vi "ContinuousStrobeSample.vi"() -> ()   [LabVIEW 2015]
panel:
  in  "Continuous \nStrobe Delay":i32
  out "Spectrum of the first Spectrometer":cluster{"Y":dbl[], "Y":dbl[]}[](graph)
  in  "stop":bool
  in  "Enter the \nInetegration Time":i32
  in  "Start":bool=TRUE
  out "Number of Spectrometers":i32
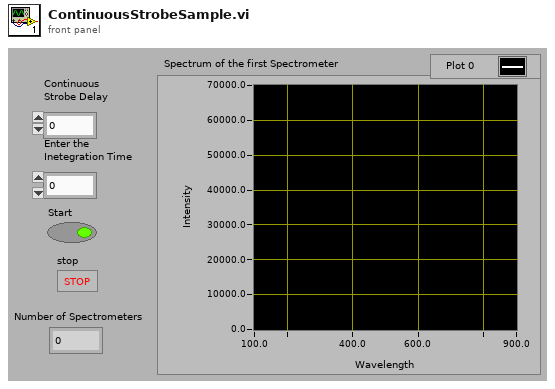
[diagram p1: front panel]
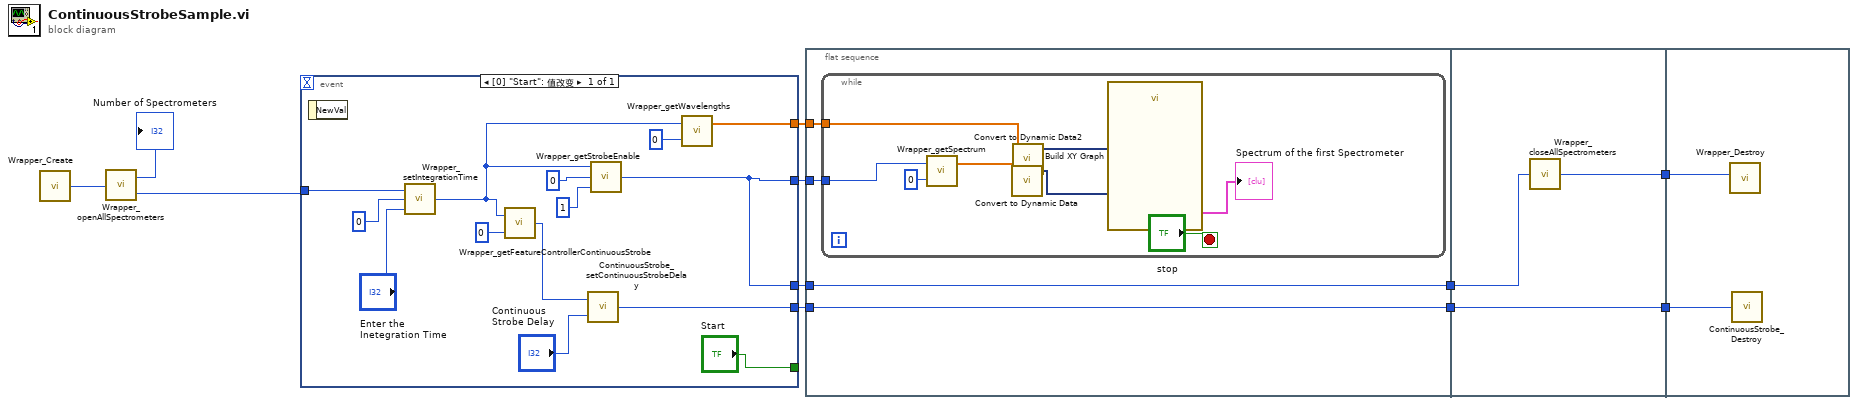
[diagram p0: block diagram]
diagram:
  n1 = call "Wrapper_Create.vi"() -> ("Wrapper"=w2:u32)
  n2 = call "Wrapper_openAllSpectrometers.vi"("Wrapper In"=w2) -> ("Number of Spectrometers"=→"Number of Spectrometers":i32, "Wrapper Out"=w1:u32)
  n3 = event shown="[0] \"Start\": 值改变" {
    selector: _ -> [_]
    dyn-events: _ -> [_]
    timeout: _ -> [_]
    tunnel: ["Start"] -> _
    tunnel: w1 -> [w22]
    tunnel: [w13] -> w10
    tunnel: [w21] -> w9
    tunnel: [w13] -> w7
    tunnel: [w12] -> w3
    event "Start": Value Change {
      n4 = event-data() -> ()  [unwired: 1 in, 1 out]
      n5 = call "Wrapper_setIntegrationTime.vi"("Integration Time"="Enter the \nInetegration Time", "Index"=0, "Wrapper In"=w22) -> ("Wrapper Out"=w16:u32)
      n6 = call "Wrapper_getFeatureControllerContinuousStrobe.vi"("Index"=0, "Wrapper"=w16) -> ("ContinuousStrobe"=w18:u32)
      n7 = call "ContinuousStrobe_setContinuousStrobeDelay.vi"("delay"="Continuous \nStrobe Delay", "ContinuousStrobe In"=w18) -> ("ContinuousStrobe Out"=w12:u32)
      n8 = call "Wrapper_getStrobeEnable.vi"("On/Off"=1, "Index"=0, "Wrapper In"=w16) -> ("Wrapper Out"=w13:u32)
      n9 = call "Wrapper_getWavelengths.vi"("Index"=0, "Wrapper"=w16) -> ("WL Values"=w21:dbl[])  [unwired: 1 out]
    }
  }
  n10 = flat-sequence {
    tunnel: w10 -> [w29]
    tunnel: w9 -> [w28]
    tunnel: [w27] -> w8
    tunnel: w7 -> [w27]
    tunnel: [w26] -> w4
    tunnel: w3 -> [w26]
    tunnel: w8 -> [w40]
    tunnel: [w39] -> w6
    tunnel: [w38] -> w5
    tunnel: w4 -> [w38]
    tunnel: w6 -> [w42]
    tunnel: w5 -> [w41]
    frame #0 {
      n11 = while {
        tunnel: w29 -> [w37]
        tunnel: w28 -> [w31]
        stop <- "stop" stop-if-true
        n12 = call "Wrapper_getSpectrum.vi"("Index"=0, "Wrapper"=w37) -> ("Spectrum Values"=w33:dbl[])  [unwired: 1 out]
        n13 = call "Convert to Dynamic Data"("Array"=w33) -> ("Dynamic Data Type"=w32:dynamicdata)  [unwired: 3 in]
        n14 = call "Convert to Dynamic Data2"("Array"=w31) -> ("Dynamic Data Type"=w30:dynamicdata)  [unwired: 3 in]
        n15 = call "Build XY Graph"("Y Input"=w32, "X Input"=w30) -> ("XY Graph"=→"Spectrum of the first Spectrometer":cluster{"Y":dbl[], "Y":dbl[]}[])  [unwired: 8 in, 1 out]
      }
    }
    frame #1 {
      n16 = call "Wrapper_closeAllSpectrometers.vi"("Wrapper In"=w40) -> ("Wrapper Out"=w39:u32)
    }
    frame #2 {
      n17 = call "Wrapper_Destroy.vi"("Wrapper"=w42) -> ()
      n18 = call "ContinuousStrobe_Destroy.vi"("ContinuousStrobe"=w41) -> ()
    }
  }
